vi "ROS_Topic_Write.vi"(2 "Msg in":string, 3 "Continuous?":bool, 4 "ROS in":T1={"topic port"=0, "Node"="", "topic"="", "type"="", "node port"=0, "error "={"status"=FALSE, "code"=0, "source"=""}, "Direction"=enum."Node", "APIs"=[], "Update (ms)"=1, "write queue"=1}) -> (1 "ROS out":T1={"topic port"=0, "Node"="", "topic"="", "type"="", "node port"=0, "error "={"status"=FALSE, "code"=0, "source"=""}, "Direction"=enum."Node", "APIs"=[], "Update (ms)"=1, "write queue"=1})   [LabVIEW 2010]
doc: "Prepends the length to Msg in before sending out the data on the specified topic. Use only for publishers and service clients. Messages need to be formatted using Message Building functionality. \n\nSetting Continuous to True will instruct the server to publish the message it received as quickly as possible, updating the message when a new ROS_Topic_Write is called."
uses:
  SubVIs/_ROSControl.ctl
  SubVIs/_ROSDirection.ctl
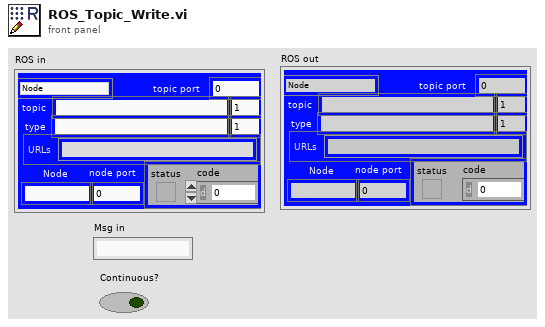
[diagram p1: front panel]
types:
  T1 = typedef "_ROSControl.ctl" = cluster{"topic port":u16, "Node":string, "topic":string, "type":string, "node port":u32, "error ":errorcluster, "Direction":T2, "APIs":string[], "Update (ms)":u16, "write queue":u16}
  T2 = typedef "_ROSDirection.ctl" = enum16{"Node", "Publisher", "Subscriber", "Service Client"}
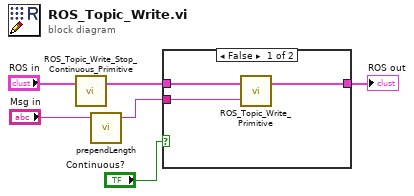
[diagram p0: block diagram]
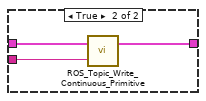
[diagram p2: hidden frame]
diagram:
  n1 = call "ROS_Topic_Write_Stop_Continuous_Primitive.vi"("ROS in"="ROS in") -> ("ROS out"=w1:T1)  [unwired: 2 in]
  n2 = call "prependLength.vi"("msg in"="Msg in") -> ("msg out"=w4:string)  [unwired: 4 in]
  n3 = case shown="False" "Continuous?" {
    tunnel: w1 -> [w9 w11]
    tunnel: [w8 w12] -> w6
    tunnel: w4 -> [w7 w10]
    frame False {
      n4 = call "ROS_Topic_Write_Primitive.vi"("Msg in"=w7, "ROS in"=w9) -> ("ROS out"=w8:T1)  [unwired: 1 in]
    }
    frame True {
      n5 = call "ROS_Topic_Write_Continuous_Primitive.vi"("Msg in"=w10, "ROS in"=w11) -> ("ROS out"=w12:T1)  [unwired: 1 in]
    }
  }
  "ROS out" <- w6
